vi "Convolute Image.vi"(0 "Image Ref (U16)":T1, 7 "Kernel":sgl[][](array[numeric])=[[1.0, 1.0, 1.0], [1.0, 1.0, 1.0], [1.0, 1.0, 1.0]] format="%.2f", 11 "Error In":errorcluster) -> (4 "Image Ref Dup":T1, 8 "Conv Image":T1, 15 "Error Out":errorcluster)   [LabVIEW 2020]
uses:
  <vilib>/vision/Image Controls.llb/IMAQ Image.ctl
  <vilib>/vision/NI_Vision_Development_Module.lvlib
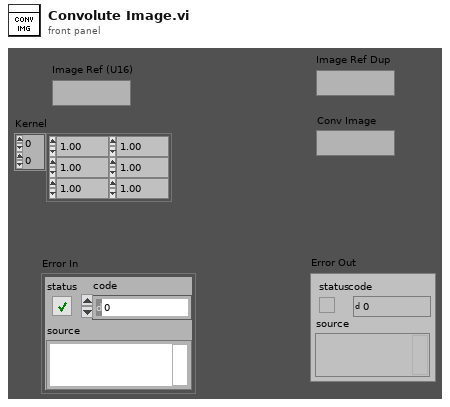
[diagram p1: front panel]
types:
  T1 = typedef "IMAQ Image.ctl" = refnum<image>
  T2 = typedef "Image Type" = u32
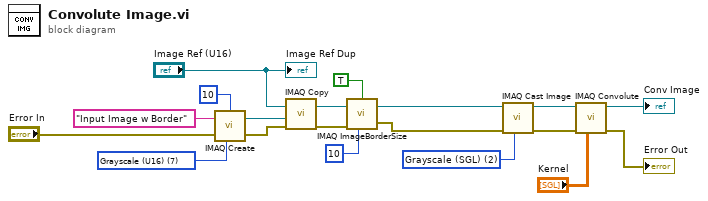
[diagram p0: block diagram]
diagram:
  w17 = T2 7 items=["Grayscale (U8)", "Grayscale (I16)", "Grayscale (SGL)", "Complex (CSG)", "RGB (U32)", "HSL (U32)", "RGB (U64)", "Grayscale (U16)"] ("Image Type")
  w19 = T2 2 items=["Grayscale (U8)", "Grayscale (I16)", "Grayscale (SGL)", "Complex (CSG)", "RGB (U32)", "HSL (U32)", "RGB (U64)", "Grayscale (U16)"] ("Image Type")
  n1 = call "IMAQ Create"("Border Size"=10, "Image Name"="Input Image w Border", "Image Type"=w17, "error in (no error)"="Error In") -> ("New Image"=w12:T1, "error out"=w14:errorcluster)  [unwired: 1 in]
  n2 = call "IMAQ Copy"("error in (no error)"=w14, "Image Dst"=w12, "Image Src"="Image Ref (U16)") -> ("error out"=w7:errorcluster, "Image Dst Out"=w11:T1)  [unwired: 3 in]
  n3 = call "IMAQ ImageBorderSize"("Get/Set Status? (Set)"=TRUE, "Image"=w11, "Image border size in"=10, "error in (no error)"=w7) -> ("Image Out"=w9:T1, "error out"=w5:errorcluster)  [unwired: 1 out]
  n4 = call "IMAQ Cast Image"("Image Type"=w19, "error in (no error)"=w5, "Image Src"=w9) -> ("error out"=w4:errorcluster, "Image Dst Out"=w18:T1)  [unwired: 7 in]
  n5 = call "IMAQ Convolute"("Kernel"="Kernel", "error in (no error)"=w4, "Image Src"=w18) -> ("error out"=→"Error Out":errorcluster, "Image Dst Out"=→"Conv Image":T1)  [unwired: 7 in]
  "Image Ref Dup" <- "Image Ref (U16)"
